vi "Get_Info_String.vi"(0 "ArrayIn":u8[](array[numeric])=[0, 0, 0, 0, 0, 0, 0, 0, 0, 0, 0, 0, 0, 0, 0, 0, 0, 0, 0, 0, 0, 0, 0, 0, 0, 0, 0, 0, 0, 0, 0, 0, 0, 0, 0, 0, 0, 0, 0, 0, 0, 0, 0, 0, 0, 0, 0, 0, 0, 0, 0, 0, 0, 0, 0, 0, 0, 0, 0, 0, 0, 0, 0, 0, 0, 0, 0, 0, 0, 0, 0, 0, 0, 0, 0, 0, 0, 0, 0, 0, 0, 0, 0, 0, 0, 0, 0, 0, 0, 0, 0, 0, 0, 0, 0, 0, 0, 0, 0, 0, 0, 0, 0, 0, 0, 0, 0, 0, 0, 0, 0, 0, 0, 0, 0, 0, 0, 0, 0, 0, 0, 0, 0, 0, 0, 0, 0, 0, 0, 0, 0, 0, 0, 0, 0, 0, 0, 0, 0, 0, 0, 0] format="0x%x", 1 "确定按钮":bool) -> (2 "bfArray":bool[][](array[boolean]), 3 "mu08ArrayOutSize":u8, 4 "strArrayOut":string[](array[string]), 5 "ValveBoolOutArray":string[][](array[string]), 6 "strValueOut":string[](array[string]), 7 "strValueOut 2":string[](array[string]))   [LabVIEW 2011]
panel:
  out "mbfArrayMotorState":string[](array[string])
  out "bfArrayActuator3":bool[](array[boolean])=[FALSE, FALSE, TRUE, FALSE, FALSE, FALSE, FALSE, FALSE, FALSE, FALSE, FALSE, FALSE, FALSE, FALSE, FALSE, FALSE, FALSE, FALSE, FALSE, FALSE, FALSE, FALSE, FALSE, FALSE, FALSE, FALSE, FALSE, FALSE, FALSE, FALSE, FALSE, FALSE]
  out "bfArrayHeater":bool[](array[boolean])
  out "bfArrayPump":bool[](array[boolean])
  out "bfArrayActuator2":bool[](array[boolean])
  out "bfArrayActuator1":bool[](array[boolean])=[FALSE, FALSE, FALSE, FALSE, FALSE, FALSE, FALSE, TRUE, FALSE, FALSE, FALSE, FALSE, FALSE, FALSE, FALSE, FALSE, FALSE, FALSE, FALSE, FALSE, FALSE, FALSE, FALSE, FALSE, FALSE, FALSE, FALSE, FALSE, FALSE, FALSE, FALSE, FALSE]
  out "bfArrayValue2":bool[](array[boolean])
  out "bfArrayValue1":bool[](array[boolean])
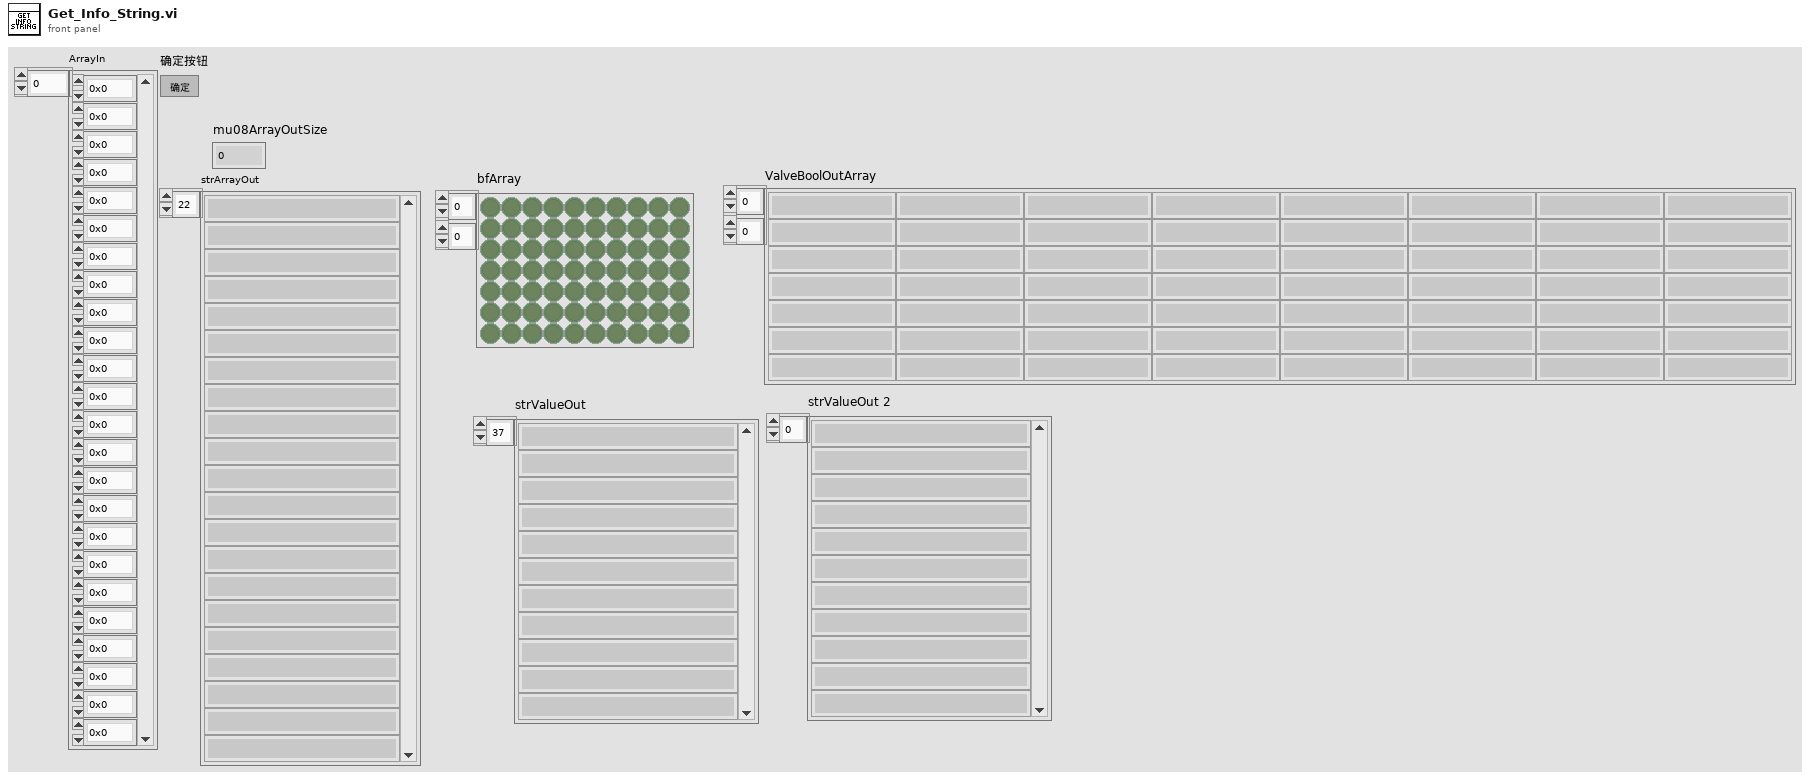
[diagram p1: front panel]
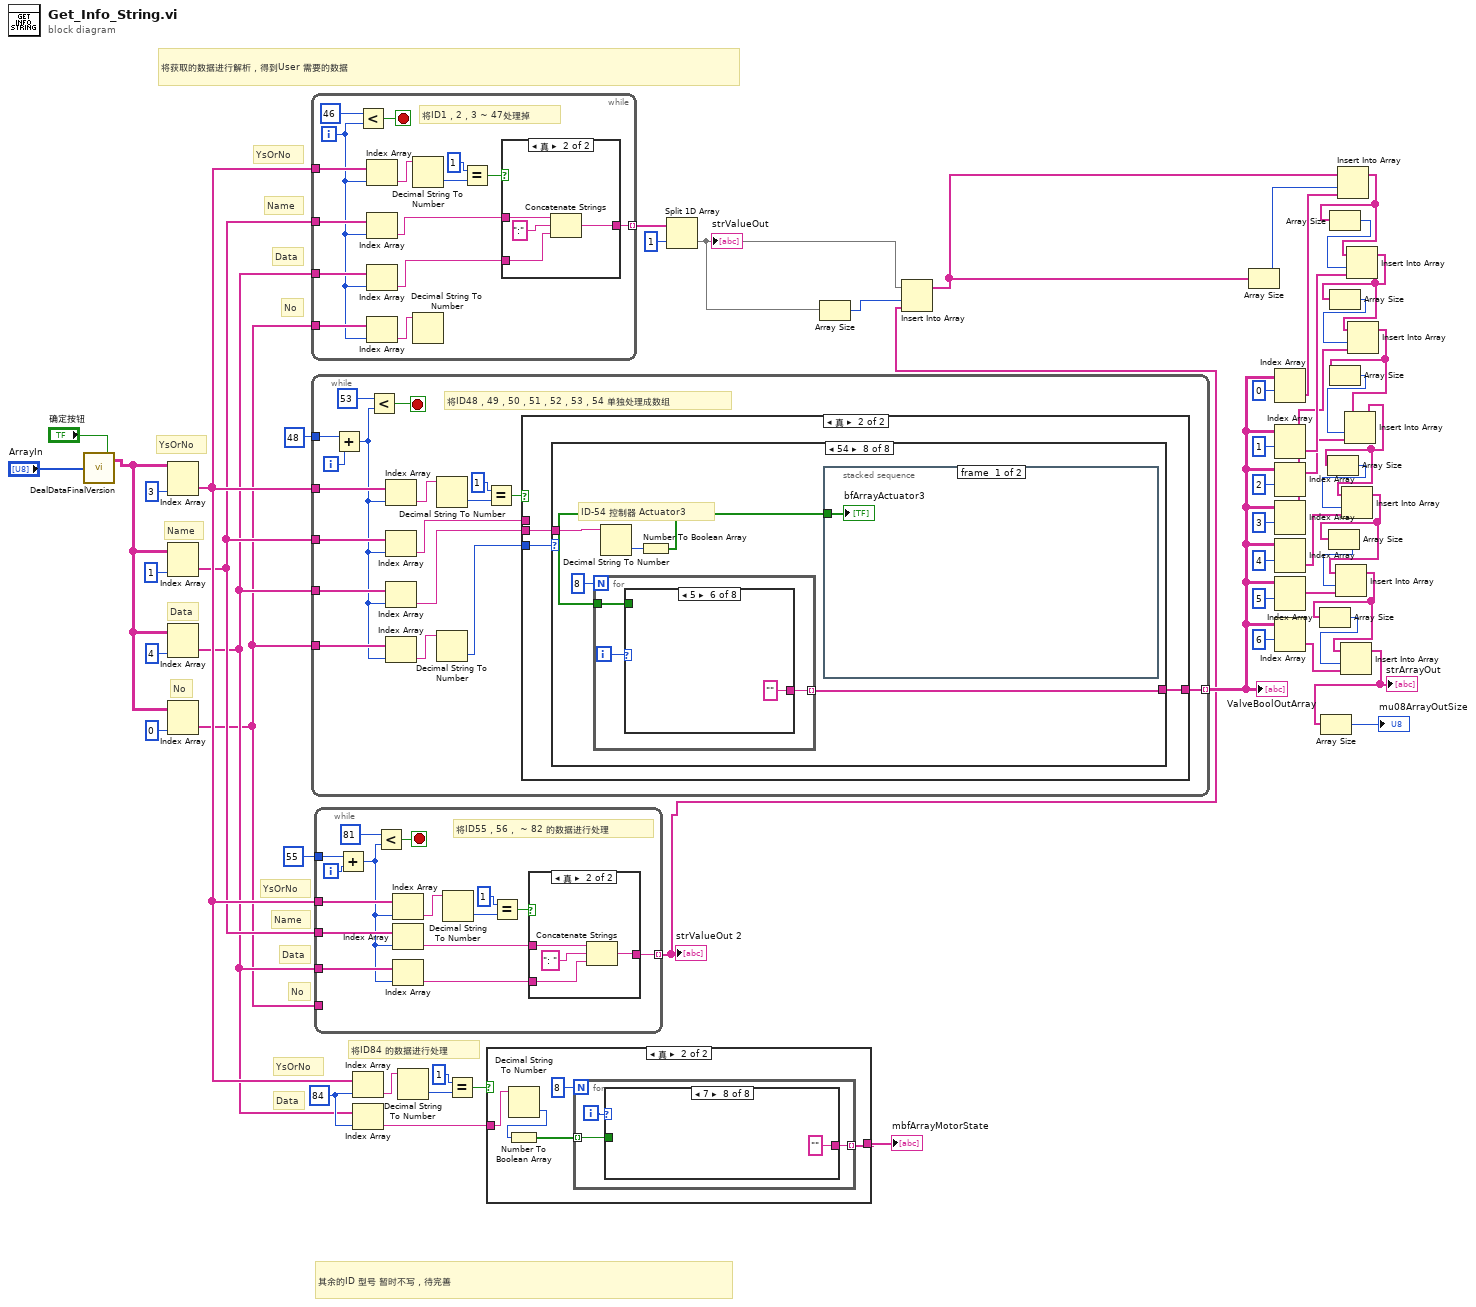
[diagram p0: block diagram]
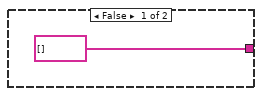
[diagram p2: hidden frame]
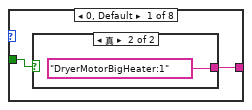
[diagram p3: hidden frame]
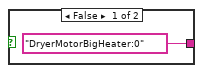
[diagram p4: hidden frame]
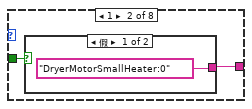
[diagram p5: hidden frame]
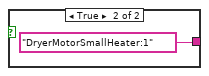
[diagram p6: hidden frame]
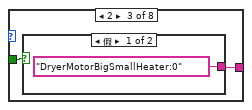
[diagram p7: hidden frame]
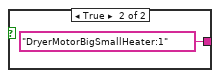
[diagram p8: hidden frame]
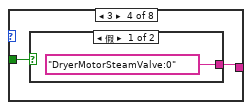
[diagram p9: hidden frame]
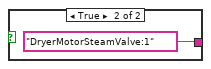
[diagram p10: hidden frame]
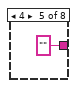
[diagram p11: hidden frame]
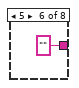
[diagram p12: hidden frame]
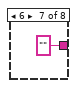
[diagram p13: hidden frame]
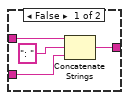
[diagram p14: hidden frame]
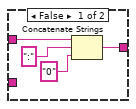
[diagram p15: hidden frame]
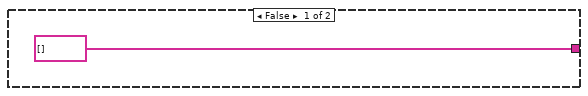
[diagram p16: hidden frame]
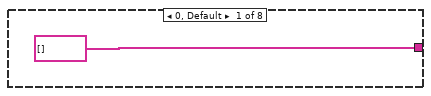
[diagram p17: hidden frame]
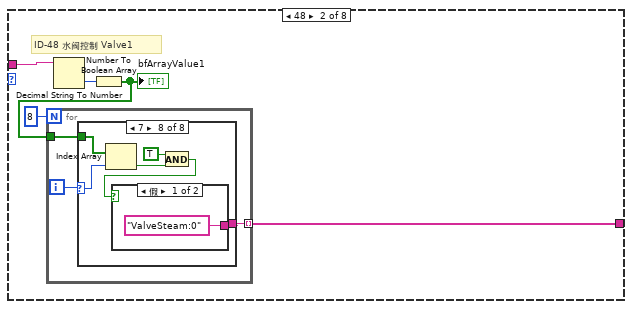
[diagram p18: hidden frame]
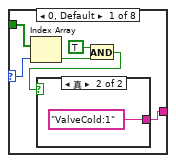
[diagram p19: hidden frame]
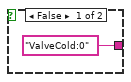
[diagram p20: hidden frame]
diagram:
  w46 = 84 ("索引")
  # "将获取的数据进行解析，得到User 需要的数据"
  # "其余的ID 型号 暂时不写，待完善"
  # "Data"
  # "YsOrNo"
  # "将ID84 的数据进行处理"
  # "No"
  # "Data"
  # "Name"
  # "YsOrNo"
  # "No"
  # "Data"
  # "Name"
  # "YsOrNo"
  # "No"
  # "Data"
  # "Name"
  # "YsOrNo"
  n1 = call "DealDataFinalVersion.vi"("ArrayIn"="ArrayIn", "确定按钮"="确定按钮") -> ("输出数组"=w2:string[][])
  n2 = Index Array(array=w2, index (col)=3 ("禁用的索引 (列)")) -> (element=w43:string[])  [unwired: 1 in]
  n3 = Index Array(array=w2, index (col)=1 ("禁用的索引 (列)")) -> (element=w42:string[])  [unwired: 1 in]
  n4 = Index Array(array=w2, index (col)=4 ("禁用的索引 (列)")) -> (element=w41:string[])  [unwired: 1 in]
  n5 = Index Array(array=w2, index (col)=0 ("禁用的索引 (列)")) -> (element=w40:string[])  [unwired: 1 in]
  n6 = while {
    tunnel: w43 -> [w69]
    tunnel: w42 -> [w65]
    tunnel: w41 -> [w64]
    tunnel: w40 -> [w63]
    tunnel: [w57] -> w38 mode=indexing
    i -> [w62]
    stop <- w71 stop-if-true
    # "将ID1，2，3 ~ 47处理掉"
    n7 = Less?(x=46, y=w62) -> (x < y?=w71:bool)
    n8 = Index Array(array=w69, index=w62) -> (element=w66:string)
    n9 = Index Array(array=w65, index=w62) -> (element=w58:string)
    n10 = Index Array(array=w64, index=w62) -> (element=w59:string)
    n11 = Index Array(array=w63, index=w62) -> (element=w60:string)
    n12 = Decimal String To Number(string=w66) -> (number=w68:i32)  [unwired: 2 in, 1 out]
    n13 = Decimal String To Number(string=w60) -> ()  [unwired: 2 in, 2 out]
    n14 = Equal?(x=1, y=w68) -> (x = y?=w61:bool)
    n15 = case shown="真" w61 {
      tunnel: w59 -> [_ w77]
      tunnel: w58 -> [w74 w79]
      tunnel: [w72 w76] -> w57
      frame False {
        n16 = Concatenate Strings(w74, ":" ("字符串"), "0" ("字符串")) -> (w72:string)
      }
      frame True {
        n17 = Concatenate Strings(w79, ":" ("字符串"), w77) -> (w76:string)
      }
    }
  }
  n18 = while {
    tunnel: w43 -> [w96]
    tunnel: w42 -> [w91]
    tunnel: w41 -> [w89]
    tunnel: w40 -> [w87]
    tunnel: 48 ("x") -> [w84]
    tunnel: [w80] -> w25 mode=indexing
    i -> [w83]
    stop <- w97 stop-if-true
    # "将ID48，49，50，51，52，53，54 单独处理成数组"
    n19 = Add(x=w84, y=w83) -> (x+y=w82:i32)
    n20 = Less?(x=53, y=w82) -> (x < y?=w97:bool)
    n21 = Index Array(array=w96, index=w82) -> (element=w95:string)
    n22 = Index Array(array=w91, index=w82) -> (element=w90:string)
    n23 = Index Array(array=w89, index=w82) -> (element=w88:string)
    n24 = Index Array(array=w87, index=w82) -> (element=w86:string)
    n25 = Decimal String To Number(string=w95) -> (number=w94:i32)  [unwired: 2 in, 1 out]
    n26 = Decimal String To Number(string=w86) -> (number=w81:i32)  [unwired: 2 in, 1 out]
    n27 = Equal?(x=1, y=w94) -> (x = y?=w92:bool)
    n28 = case shown="真" w92 {
      tunnel: w90 -> [_ _]
      tunnel: w88 -> [_ w100]
      tunnel: w81 -> [_ w101]
      tunnel: [string[] [] w99] -> w80
      frame False {
      }
      frame True {
        n29 = case shown="54" w101 {
          tunnel: w100 -> [_ w104 w176 w227 w299 w371 w408 w460]
          tunnel: [string[] [] w103 w175 w226 w298 w370 w407 w459] -> w99
          frame 0, Default {
          }
          frame 48 {
            # "ID-48 水阀控制 Valve1"
            n30 = Decimal String To Number(string=w104) -> (number=w105:i32)  [unwired: 2 in, 1 out]
            n31 = Number To Boolean Array(number=w105) -> (Boolean array=w107:bool[])
            "bfArrayValue1" <- w107
            n32 = for {
              N: 8 -> [_]
              tunnel: w107 -> [w109]
              tunnel: [w108] -> w103 mode=indexing
              i -> [w110]
              n33 = case shown="7" w110 {
                selector: w110 -> [w116 w121 w129 w137 w145 w153 w161 w169]
                tunnel: w109 -> [w115 w120 w128 w136 w144 w152 w160 w168]
                tunnel: [w111 w119 w127 w135 w143 w151 w159 w167] -> w108
                frame 0, Default {
                  n34 = Index Array(array=w115, index=w116) -> (element=w114:bool)
                  n35 = And(x=TRUE, y=w114) -> (x .and. y?=w112:bool)
                  n36 = case shown="真" w112 {
                    tunnel: ["ValveCold:0" "ValveCold:1"] -> w111
                    frame False {
                    }
                    frame True {
                    }
                  }
                }
                frame 1 {
                  n37 = Index Array(array=w120, index=w121) -> (element=w124:bool)
                  n38 = And(x=TRUE, y=w124) -> (x .and. y?=w122:bool)
                  n39 = case shown="真" w122 {
                    tunnel: ["ValveHot:0" "ValveHot:1"] -> w119
                    frame False {
                    }
                    frame True {
                    }
                  }
                }
                frame 2 {
                  n40 = Index Array(array=w128, index=w129) -> (element=w132:bool)
                  n41 = And(x=TRUE, y=w132) -> (x .and. y?=w130:bool)
                  n42 = case shown="真" w130 {
                    tunnel: ["ValvePre:0" "ValvePre:1"] -> w127
                    frame False {
                    }
                    frame True {
                    }
                  }
                }
                frame 3 {
                  n43 = Index Array(array=w136, index=w137) -> (element=w140:bool)
                  n44 = And(x=TRUE, y=w140) -> (x .and. y?=w138:bool)
                  n45 = case shown="真" w138 {
                    tunnel: ["WaterShot:0" "WaterShot:1"] -> w135
                    frame False {
                    }
                    frame True {
                    }
                  }
                }
                frame 4 {
                  n46 = Index Array(array=w144, index=w145) -> (element=w148:bool)
                  n47 = And(x=TRUE, y=w148) -> (x .and. y?=w146:bool)
                  n48 = case shown="假" w146 {
                    tunnel: ["WaterBleach:0" "WaterBleach:1"] -> w143
                    frame False {
                    }
                    frame True {
                    }
                  }
                }
                frame 5 {
                  n49 = Index Array(array=w152, index=w153) -> (element=w156:bool)
                  n50 = And(x=TRUE, y=w156) -> (x .and. y?=w154:bool)
                  n51 = case shown="假" w154 {
                    tunnel: ["ValveDry:0" "ValveDry:1"] -> w151
                    frame False {
                    }
                    frame True {
                    }
                  }
                }
                frame 6 {
                  n52 = Index Array(array=w160, index=w161) -> (element=w164:bool)
                  n53 = And(x=TRUE, y=w164) -> (x .and. y?=w162:bool)
                  n54 = case shown="假" w162 {
                    tunnel: ["ValveMist:0" "ValveMist:1"] -> w159
                    frame False {
                    }
                    frame True {
                    }
                  }
                }
                frame 7 {
                  n55 = Index Array(array=w168, index=w169) -> (element=w172:bool)
                  n56 = And(x=TRUE, y=w172) -> (x .and. y?=w170:bool)
                  n57 = case shown="假" w170 {
                    tunnel: ["ValveSteam:0" "ValveSteam:1"] -> w167
                    frame False {
                    }
                    frame True {
                    }
                  }
                }
              }
            }
          }
          frame 49 {
            # "ID-49 水阀控制 Valve2"
            n58 = Decimal String To Number(string=w176) -> (number=w177:i32)  [unwired: 2 in, 1 out]
            n59 = Number To Boolean Array(number=w177) -> (Boolean array=w179:bool[])
            "bfArrayValue2" <- w179
            n60 = for {
              N: 8 -> [_]
              tunnel: w179 -> [w181]
              tunnel: [w180] -> w175 mode=indexing
              i -> [w182]
              n61 = case shown="7" w182 {
                selector: w182 -> [w188 _ w194 w202 w210 w218 _ _]
                tunnel: w181 -> [w187 _ w193 w201 w209 w217 _ _]
                tunnel: [w183 "" w192 w200 w208 w216 "" ""] -> w180
                frame 0, Default {
                  n62 = Index Array(array=w187, index=w188) -> (element=w186:bool)
                  n63 = And(x=TRUE, y=w186) -> (x .and. y?=w184:bool)
                  n64 = case shown="真" w184 {
                    tunnel: ["ValveChange:0" "ValveChange:1"] -> w183
                    frame False {
                    }
                    frame True {
                    }
                  }
                }
                frame 1 {
                }
                frame 2 {
                  n65 = Index Array(array=w193, index=w194) -> (element=w197:bool)
                  n66 = And(x=TRUE, y=w197) -> (x .and. y?=w195:bool)
                  n67 = case shown="假" w195 {
                    tunnel: ["ValveSoftener:0" "ValveSoftener:1"] -> w192
                    frame False {
                    }
                    frame True {
                    }
                  }
                }
                frame 3 {
                  n68 = Index Array(array=w201, index=w202) -> (element=w205:bool)
                  n69 = And(x=TRUE, y=w205) -> (x .and. y?=w203:bool)
                  n70 = case shown="真" w203 {
                    tunnel: ["ValueFilter:0" "ValueFilter:1"] -> w200
                    frame False {
                    }
                    frame True {
                    }
                  }
                }
                frame 4 {
                  n71 = Index Array(array=w209, index=w210) -> (element=w213:bool)
                  n72 = And(x=TRUE, y=w213) -> (x .and. y?=w211:bool)
                  n73 = case shown="假" w211 {
                    tunnel: ["ValveActiveWash:0" "ValveActiveWash:1"] -> w208
                    frame False {
                    }
                    frame True {
                    }
                  }
                }
                frame 5 {
                  n74 = Index Array(array=w217, index=w218) -> (element=w221:bool)
                  n75 = And(x=TRUE, y=w221) -> (x .and. y?=w219:bool)
                  n76 = case shown="真" w219 {
                    tunnel: ["WaterBleach: 0" "WaterBleach:1"] -> w216
                    frame False {
                    }
                    frame True {
                    }
                  }
                }
                frame 6 {
                }
                frame 7 {
                }
              }
            }
          }
          frame 50 {
            # "ID-50 控制器 Actuator1"
            n77 = Decimal String To Number(string=w227) -> (number=w229:i32)  [unwired: 2 in, 1 out]
            n78 = Number To Boolean Array(number=w229) -> (Boolean array=w228:bool[])
            "bfArrayActuator1" <- w228
            n79 = for {
              N: 8 -> [_]
              tunnel: w228 -> [w232]
              tunnel: [w231] -> w226 mode=indexing
              i -> [w233]
              n80 = case shown="0, 默认" w233 {
                selector: w233 -> [w239 w244 w252 w260 w268 w276 w284 w292]
                tunnel: w232 -> [w238 w243 w251 w259 w267 w275 w283 w291]
                tunnel: [w234 w242 w250 w258 w266 w274 w282 w290] -> w231
                frame 0, Default {
                  n81 = Index Array(array=w238, index=w239) -> (element=w237:bool)
                  n82 = And(x=TRUE, y=w237) -> (x .and. y?=w235:bool)
                  n83 = case shown="真" w235 {
                    tunnel: ["MotorAC:0" "MotorAC:1"] -> w234
                    frame False {
                    }
                    frame True {
                    }
                  }
                }
                frame 1 {
                  n84 = Index Array(array=w243, index=w244) -> (element=w247:bool)
                  n85 = And(x=TRUE, y=w247) -> (x .and. y?=w245:bool)
                  n86 = case shown="假" w245 {
                    tunnel: ["MotorFan:0" "MotorFan:1"] -> w242
                    frame False {
                    }
                    frame True {
                    }
                  }
                }
                frame 2 {
                  n87 = Index Array(array=w251, index=w252) -> (element=w255:bool)
                  n88 = And(x=TRUE, y=w255) -> (x .and. y?=w253:bool)
                  n89 = case shown="真" w253 {
                    tunnel: ["MotorClutch:0" "MotorClutch:1"] -> w250
                    frame False {
                    }
                    frame True {
                    }
                  }
                }
                frame 3 {
                  n90 = Index Array(array=w259, index=w260) -> (element=w263:bool)
                  n91 = And(x=TRUE, y=w263) -> (x .and. y?=w261:bool)
                  n92 = case shown="假" w261 {
                    tunnel: ["DoorLock:0" "DoorLock:1"] -> w258
                    frame False {
                    }
                    frame True {
                    }
                  }
                }
                frame 4 {
                  n93 = Index Array(array=w267, index=w268) -> (element=w271:bool)
                  n94 = And(x=TRUE, y=w271) -> (x .and. y?=w269:bool)
                  n95 = case shown="假" w269 {
                    tunnel: ["MotorAutoDetergent:0" "MotorAutoDetergent:1"] -> w266
                    frame False {
                    }
                    frame True {
                    }
                  }
                }
                frame 5 {
                  n96 = Index Array(array=w275, index=w276) -> (element=w279:bool)
                  n97 = And(x=TRUE, y=w279) -> (x .and. y?=w277:bool)
                  n98 = case shown="真" w277 {
                    tunnel: ["MotorAutoRinse:0" "MotorAutoRinse:1"] -> w274
                    frame False {
                    }
                    frame True {
                    }
                  }
                }
                frame 6 {
                  n99 = Index Array(array=w283, index=w284) -> (element=w287:bool)
                  n100 = And(x=TRUE, y=w287) -> (x .and. y?=w285:bool)
                  n101 = case shown="假" w285 {
                    tunnel: ["SSR:0" "SSR:1"] -> w282
                    frame False {
                    }
                    frame True {
                    }
                  }
                }
                frame 7 {
                  n102 = Index Array(array=w291, index=w292) -> (element=w295:bool)
                  n103 = And(x=TRUE, y=w295) -> (x .and. y?=w293:bool)
                  n104 = case shown="假" w293 {
                    tunnel: ["MainRelay:0" "MainRelay:1"] -> w290
                    frame False {
                    }
                    frame True {
                    }
                  }
                }
              }
            }
          }
          frame 51 {
            # "ID-51 控制器 Actuator2"
            n105 = Decimal String To Number(string=w299) -> (number=w301:i32)  [unwired: 2 in, 1 out]
            n106 = Number To Boolean Array(number=w301) -> (Boolean array=w300:bool[])
            "bfArrayActuator2" <- w300
            n107 = for {
              N: 8 -> [_]
              tunnel: w300 -> [w304]
              tunnel: [w303] -> w298 mode=indexing
              i -> [w305]
              n108 = case shown="7" w305 {
                selector: w305 -> [w311 w316 w324 w332 w340 w348 w356 w364]
                tunnel: w304 -> [w310 w315 w323 w331 w339 w347 w355 w363]
                tunnel: [w306 w314 w322 w330 w338 w346 w354 w362] -> w303
                frame 0, Default {
                  n109 = Index Array(array=w310, index=w311) -> (element=w309:bool)
                  n110 = And(x=TRUE, y=w309) -> (x .and. y?=w307:bool)
                  n111 = case shown="假" w307 {
                    tunnel: ["MotorDistributor:0" "MotorDistributor:1"] -> w306
                    frame False {
                    }
                    frame True {
                    }
                  }
                }
                frame 1 {
                  n112 = Index Array(array=w315, index=w316) -> (element=w319:bool)
                  n113 = And(x=TRUE, y=w319) -> (x .and. y?=w317:bool)
                  n114 = case shown="真" w317 {
                    tunnel: ["TurbiditySensorOnOff:0" "TurbiditySensorOnOff:1"] -> w314
                    frame False {
                    }
                    frame True {
                    }
                  }
                }
                frame 2 {
                  n115 = Index Array(array=w323, index=w324) -> (element=w327:bool)
                  n116 = And(x=TRUE, y=w327) -> (x .and. y?=w325:bool)
                  n117 = case shown="假" w325 {
                    tunnel: ["ActuatorDry:0" "ActuatorDry:1"] -> w322
                    frame False {
                    }
                    frame True {
                    }
                  }
                }
                frame 3 {
                  n118 = Index Array(array=w331, index=w332) -> (element=w335:bool)
                  n119 = And(x=TRUE, y=w335) -> (x .and. y?=w333:bool)
                  n120 = case shown="真" w333 {
                    tunnel: ["ActuatorDoorOpen:0" "ActuatorDoorOpen:1"] -> w330
                    frame False {
                    }
                    frame True {
                    }
                  }
                }
                frame 4 {
                  n121 = Index Array(array=w339, index=w340) -> (element=w343:bool)
                  n122 = And(x=TRUE, y=w343) -> (x .and. y?=w341:bool)
                  n123 = case shown="真" w341 {
                    tunnel: ["VaneCW:0" "VaneCW:1"] -> w338
                    frame False {
                    }
                    frame True {
                    }
                  }
                }
                frame 5 {
                  n124 = Index Array(array=w347, index=w348) -> (element=w351:bool)
                  n125 = And(x=TRUE, y=w351) -> (x .and. y?=w349:bool)
                  n126 = case shown="真" w349 {
                    tunnel: ["VaneCCW:0" "VaneCCW:1"] -> w346
                    frame False {
                    }
                    frame True {
                    }
                  }
                }
                frame 6 {
                  n127 = Index Array(array=w355, index=w356) -> (element=w359:bool)
                  n128 = And(x=TRUE, y=w359) -> (x .and. y?=w357:bool)
                  n129 = case shown="真" w357 {
                    tunnel: ["IVTPower1:0" "IVTPower1:1"] -> w354
                    frame False {
                    }
                    frame True {
                    }
                  }
                }
                frame 7 {
                  n130 = Index Array(array=w363, index=w364) -> (element=w367:bool)
                  n131 = And(x=TRUE, y=w367) -> (x .and. y?=w365:bool)
                  n132 = case shown="真" w365 {
                    tunnel: ["IVTPower2:0" "IVTPower2:1"] -> w362
                    frame False {
                    }
                    frame True {
                    }
                  }
                }
              }
            }
          }
          frame 52 {
            # "ID-52 控制阀 Pump"
            n133 = Decimal String To Number(string=w371) -> (number=w373:i32)  [unwired: 2 in, 1 out]
            n134 = Number To Boolean Array(number=w373) -> (Boolean array=w372:bool[])
            "bfArrayPump" <- w372
            n135 = for {
              N: 8 -> [_]
              tunnel: w372 -> [w376]
              tunnel: [w375] -> w370 mode=indexing
              i -> [w377]
              n136 = case shown="7" w377 {
                selector: w377 -> [w383 w388 w396 _ _ _ _ _]
                tunnel: w376 -> [w382 w387 w395 _ _ _ _ _]
                tunnel: [w378 w386 w394 "" "" "" "" ""] -> w375
                frame 0, Default {
                  n137 = Index Array(array=w382, index=w383) -> (element=w381:bool)
                  n138 = And(x=TRUE, y=w381) -> (x .and. y?=w379:bool)
                  n139 = case shown="假" w379 {
                    tunnel: ["PumpDrain:0" "PumpDrain:1"] -> w378
                    frame False {
                    }
                    frame True {
                    }
                  }
                }
                frame 1 {
                  n140 = Index Array(array=w387, index=w388) -> (element=w391:bool)
                  n141 = And(x=TRUE, y=w391) -> (x .and. y?=w389:bool)
                  n142 = case shown="假" w389 {
                    tunnel: ["PumpCircuration:0" "PumpCircuration:1"] -> w386
                    frame False {
                    }
                    frame True {
                    }
                  }
                }
                frame 2 {
                  n143 = Index Array(array=w395, index=w396) -> (element=w399:bool)
                  n144 = And(x=TRUE, y=w399) -> (x .and. y?=w397:bool)
                  n145 = case shown="假" w397 {
                    tunnel: ["PumpBubble:0" "PumpBubble:1"] -> w394
                    frame False {
                    }
                    frame True {
                    }
                  }
                }
                frame 3 {
                }
                frame 4 {
                }
                frame 5 {
                }
                frame 6 {
                }
                frame 7 {
                }
              }
            }
          }
          frame 53 {
            # "ID-53 加热器控制 Heater"
            n146 = Decimal String To Number(string=w408) -> (number=w409:i32)  [unwired: 2 in, 1 out]
            n147 = Number To Boolean Array(number=w409) -> (Boolean array=w411:bool[])
            "bfArrayHeater" <- w411
            n148 = for {
              N: 8 -> [_]
              tunnel: w411 -> [w413]
              tunnel: [w412] -> w407 mode=indexing
              i -> [w414]
              n149 = case shown="7" w414 {
                selector: w414 -> [w420 w425 w433 w441 w449 _ _ _]
                tunnel: w413 -> [w419 w424 w432 w440 w448 _ _ _]
                tunnel: [w415 w423 w431 w439 w447 "" "" ""] -> w412
                frame 0, Default {
                  n150 = Index Array(array=w419, index=w420) -> (element=w418:bool)
                  n151 = And(x=TRUE, y=w418) -> (x .and. y?=w416:bool)
                  n152 = case shown="真" w416 {
                    tunnel: ["HeaterWash:0" "HeaterWash:1"] -> w415
                    frame False {
                    }
                    frame True {
                    }
                  }
                }
                frame 1 {
                  n153 = Index Array(array=w424, index=w425) -> (element=w428:bool)
                  n154 = And(x=TRUE, y=w428) -> (x .and. y?=w426:bool)
                  n155 = case shown="真" w426 {
                    tunnel: ["HeaterDry:0" "HeaterDry:1"] -> w423
                    frame False {
                    }
                    frame True {
                    }
                  }
                }
                frame 2 {
                  n156 = Index Array(array=w432, index=w433) -> (element=w436:bool)
                  n157 = And(x=TRUE, y=w436) -> (x .and. y?=w434:bool)
                  n158 = case shown="真" w434 {
                    tunnel: ["HeaterSteam:0" "HeaterSteam:1"] -> w431
                    frame False {
                    }
                    frame True {
                    }
                  }
                }
                frame 3 {
                  n159 = Index Array(array=w440, index=w441) -> (element=w444:bool)
                  n160 = And(x=TRUE, y=w444) -> (x .and. y?=w442:bool)
                  n161 = case shown="假" w442 {
                    tunnel: ["HeaterDryerLarge:0" "HeaterDryerLarge:1"] -> w439
                    frame False {
                    }
                    frame True {
                    }
                  }
                }
                frame 4 {
                  n162 = Index Array(array=w448, index=w449) -> (element=w452:bool)
                  n163 = And(x=TRUE, y=w452) -> (x .and. y?=w450:bool)
                  n164 = case shown="假" w450 {
                    tunnel: ["HeaterDryerSmall:0" "HeaterDryerSmall:1"] -> w447
                    frame False {
                    }
                    frame True {
                    }
                  }
                }
                frame 5 {
                }
                frame 6 {
                }
                frame 7 {
                }
              }
            }
          }
          frame 54 {
            # "ID-54 控制器 Actuator3"
            n165 = Decimal String To Number(string=w460) -> (number=w461:i32)  [unwired: 2 in, 1 out]
            n166 = Number To Boolean Array(number=w461) -> (Boolean array=w458:bool[])
            n167 = for {
              N: 8 -> [_]
              tunnel: w458 -> [w473]
              tunnel: [w472] -> w459 mode=indexing
              i -> [w474]
              n168 = case shown="5" w474 {
                selector: w474 -> [w480 w485 w493 w501 _ _ w511 w519]
                tunnel: w473 -> [w479 w484 w492 w500 _ _ w510 w518]
                tunnel: [w475 w483 w491 w499 "" "" w509 w517] -> w472
                frame 0, Default {
                  n169 = Index Array(array=w479, index=w480) -> (element=w478:bool)
                  n170 = And(x=TRUE, y=w478) -> (x .and. y?=w476:bool)
                  n171 = case shown="假" w476 {
                    tunnel: ["MotorCW:0" "MotorCW:1"] -> w475
                    frame False {
                    }
                    frame True {
                    }
                  }
                }
                frame 1 {
                  n172 = Index Array(array=w484, index=w485) -> (element=w488:bool)
                  n173 = And(x=TRUE, y=w488) -> (x .and. y?=w486:bool)
                  n174 = case shown="假" w486 {
                    tunnel: ["MotorCCW:0" "MotorCCW:1"] -> w483
                    frame False {
                    }
                    frame True {
                    }
                  }
                }
                frame 2 {
                  n175 = Index Array(array=w492, index=w493) -> (element=w496:bool)
                  n176 = And(x=TRUE, y=w496) -> (x .and. y?=w494:bool)
                  n177 = case shown="真" w494 {
                    tunnel: ["MotorDirection:0" "MotorDirection:1"] -> w491
                    frame False {
                    }
                    frame True {
                    }
                  }
                }
                frame 3 {
                  n178 = Index Array(array=w500, index=w501) -> (element=w504:bool)
                  n179 = And(x=TRUE, y=w504) -> (x .and. y?=w502:bool)
                  n180 = case shown="真" w502 {
                    tunnel: ["Strainer:0" "Strainer:1"] -> w499
                    frame False {
                    }
                    frame True {
                    }
                  }
                }
                frame 4 {
                }
                frame 5 {
                }
                frame 6 {
                  n181 = Index Array(array=w510, index=w511) -> (element=w514:bool)
                  n182 = And(x=TRUE, y=w514) -> (x .and. y?=w512:bool)
                  n183 = case shown="假" w512 {
                    tunnel: ["AddDoor:0" "AddDoor:1"] -> w509
                    frame False {
                    }
                    frame True {
                    }
                  }
                }
                frame 7 {
                  n184 = Index Array(array=w518, index=w519) -> (element=w522:bool)
                  n185 = And(x=TRUE, y=w522) -> (x .and. y?=w520:bool)
                  n186 = case shown="假" w520 {
                    tunnel: ["AddDoorLock:0" "AddDoorLock:1"] -> w517
                    frame False {
                    }
                    frame True {
                    }
                  }
                }
              }
            }
            n187 = stacked-sequence {
              tunnel: w458 -> [w463 _]
              frame #0 {
                "bfArrayActuator3" <- w463
              }
              frame #1 {
                n188 = local read "bfArrayValue1"() -> (w464:bool[])
                n189 = local read "bfArrayValue2"() -> (w465:bool[])
                n190 = local read "bfArrayActuator1"() -> (w466:bool[])
                n191 = local read "bfArrayActuator2"() -> (w467:bool[])
                n192 = local read "bfArrayPump"() -> (w468:bool[])
                n193 = local read "bfArrayHeater"() -> (w469:bool[])
                n194 = local read "bfArrayActuator3"() -> (w470:bool[])
                n195 = Build Array(w464, w465, w466, w467, w468, w469, w470) -> (→"bfArray":bool[][])
              }
            }
          }
        }
      }
    }
  }
  "ValveBoolOutArray" <- w25
  n196 = while {
    tunnel: 55 ("x") -> [w538]
    tunnel: w43 -> [w533]
    tunnel: w42 -> [w531]
    tunnel: w41 -> [w530]
    tunnel: w40 -> [_]
    tunnel: [w525] -> w5 mode=indexing
    i -> [w537]
    stop <- w539 stop-if-true
    # "将ID55，56， ~ 82 的数据进行处理"
    n197 = Add(x=w538, y=w537) -> (x+y=w529:i32)
    n198 = Less?(x=81, y=w529) -> (x < y?=w539:bool)
    n199 = Index Array(array=w533, index=w529) -> (element=w532:string)
    n200 = Index Array(array=w531, index=w529) -> (element=w527:string)
    n201 = Index Array(array=w530, index=w529) -> (element=w526:string)
    n202 = Decimal String To Number(string=w532) -> (number=w535:i32)  [unwired: 2 in, 1 out]
    n203 = Equal?(x=1, y=w535) -> (x = y?=w528:bool)
    n204 = case shown="真" w528 {
      tunnel: w527 -> [w542 w547]
      tunnel: w526 -> [w541 w545]
      tunnel: [w540 w544] -> w525
      frame False {
        n205 = Concatenate Strings(w542, ": " ("字符串"), w541) -> (w540:string)
      }
      frame True {
        n206 = Concatenate Strings(w547, ": " ("字符串"), w545) -> (w544:string)
      }
    }
  }
  "strValueOut 2" <- w5
  n207 = Index Array(array=w43, index=w46) -> (element=w48:string)
  n208 = Index Array(array=w41, index=w46) -> (element=w45:string)
  n209 = Decimal String To Number(string=w48) -> (number=w49:i32)  [unwired: 2 in, 1 out]
  n210 = Equal?(x=1, y=w49) -> (x = y?=w47:bool)
  n211 = case shown="真" w47 {
    tunnel: w45 -> [_ w552]
    tunnel: [string[] [] w549] -> w44
    frame False {
    }
    frame True {
      n212 = Decimal String To Number(string=w552) -> (number=w551:i32)  [unwired: 2 in, 1 out]
      n213 = Number To Boolean Array(number=w551) -> (Boolean array=w550:bool[])
      n214 = for {
        N: 8 -> [_]
        tunnel: w550 -> [w555] mode=indexing
        tunnel: [w554] -> w549 mode=indexing
        i -> [w556]
        n215 = case shown="7" w556 {
          tunnel: w555 -> [w558 w562 w566 w570 _ _ _ _]
          tunnel: [w557 w561 w565 w569 "" "" "" ""] -> w554
          frame 0, Default {
            n216 = case shown="真" w558 {
              tunnel: ["DryerMotorBigHeater:0" "DryerMotorBigHeater:1"] -> w557
              frame False {
              }
              frame True {
              }
            }
          }
          frame 1 {
            n217 = case shown="假" w562 {
              tunnel: ["DryerMotorSmallHeater:0" "DryerMotorSmallHeater:1"] -> w561
              frame False {
              }
              frame True {
              }
            }
          }
          frame 2 {
            n218 = case shown="假" w566 {
              tunnel: ["DryerMotorBigSmallHeater:0" "DryerMotorBigSmallHeater:1"] -> w565
              frame False {
              }
              frame True {
              }
            }
          }
          frame 3 {
            n219 = case shown="假" w570 {
              tunnel: ["DryerMotorSteamValve:0" "DryerMotorSteamValve:1"] -> w569
              frame False {
              }
              frame True {
              }
            }
          }
          frame 4 {
          }
          frame 5 {
          }
          frame 6 {
          }
          frame 7 {
          }
        }
      }
    }
  }
  "mbfArrayMotorState" <- w44
  n220 = Split 1D Array(array=w38, index=1 ("索引")) -> (second subarray=w6:string[])  [unwired: 1 out]
  "strValueOut" <- w6
  n221 = Array Size(array=w6) -> (size(s)=w7:i32)
  n222 = Insert Into Array(array=w6, index=w7, new element=w5) -> (w4:string[])
  n223 = Array Size(array=w4) -> (size(s)=w37:i32)
  n224 = Index Array(array=w25, index (row)=0 ("索引 (行)")) -> (element=w34:string[])  [unwired: 1 in]
  n225 = Index Array(array=w25, index (row)=1 ("索引 (行)")) -> (element=w32:string[])  [unwired: 1 in]
  n226 = Index Array(array=w25, index (row)=2 ("索引 (行)")) -> (element=w22:string[])  [unwired: 1 in]
  n227 = Index Array(array=w25, index (row)=3 ("索引 (行)")) -> (element=w19:string[])  [unwired: 1 in]
  n228 = Index Array(array=w25, index (row)=4 ("索引 (行)")) -> (element=w16:string[])  [unwired: 1 in]
  n229 = Index Array(array=w25, index (row)=5 ("索引 (行)")) -> (element=w13:string[])  [unwired: 1 in]
  n230 = Index Array(array=w25, index (row)=6 ("索引 (行)")) -> (element=w10:string[])  [unwired: 1 in]
  n231 = Insert Into Array(array=w4, index=w37, new element=w34) -> (w31:string[])
  n232 = Array Size(array=w31) -> (size(s)=w33:i32)
  n233 = Insert Into Array(array=w31, index=w33, new element=w32) -> (w23:string[])
  n234 = Array Size(array=w23) -> (size(s)=w24:i32)
  n235 = Insert Into Array(array=w23, index=w24, new element=w22) -> (w20:string[])
  n236 = Array Size(array=w20) -> (size(s)=w21:i32)
  n237 = Insert Into Array(array=w20, index=w21, new element=w19) -> (w17:string[])
  n238 = Array Size(array=w17) -> (size(s)=w18:i32)
  n239 = Insert Into Array(array=w17, index=w18, new element=w16) -> (w15:string[])
  n240 = Array Size(array=w15) -> (size(s)=w14:i32)
  n241 = Insert Into Array(array=w15, index=w14, new element=w13) -> (w11:string[])
  n242 = Array Size(array=w11) -> (size(s)=w12:i32)
  n243 = Insert Into Array(array=w11, index=w12, new element=w10) -> (w9:string[])
  "strArrayOut" <- w9
  n244 = Array Size(array=w9) -> (size(s)=→"mu08ArrayOutSize":i32)
